vi "NanotecSMCPDDriver.set standby current.vi"(0 "VISA resource name":refnum<visa-resource-name>, 1 "contollerID":i32=-1, 3 "standbyCurrent [A]":dbl, 5 "error in (no error)":errorcluster) -> (14 "VISA resource name out":refnum<visa-resource-name>, 15 "contollerID out":i32=-1, 19 "error out":errorcluster)   [LabVIEW 2014, in "NanotecSMCPDDriver.lvlib"]
doc: "Sets the phase current of the motor that will be used in stand-by mode. This current will be applied when the motor is not moving."
uses:
  NanotecSMCPDDriver.lvlib
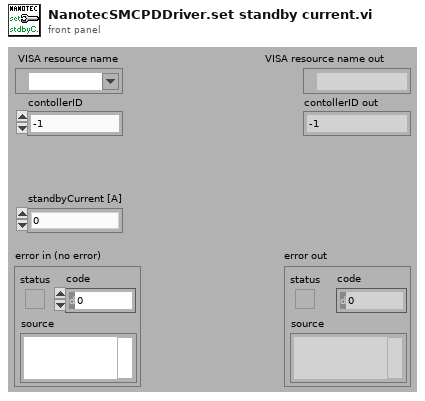
[diagram p1: front panel]
types:
  T1 = typedef "NanotecSMCPDDriver.lvlib/NanotecSMCPDDriver.hardware types.ctl" = enum16{"unknown", "PD4", "PD4Ic", "PD2Ic", "SMCI32", "SMCI47"}
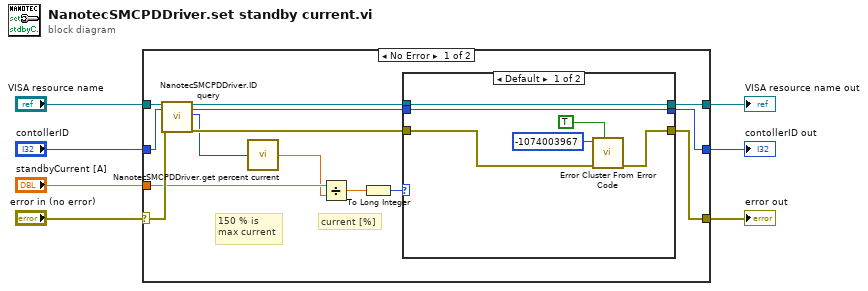
[diagram p0: block diagram]
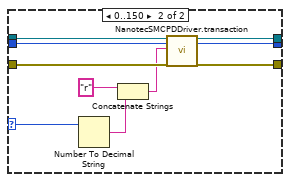
[diagram p2: hidden frame]
diagram:
  n1 = case shown="No Error" "error in (no error)" {
    selector: "error in (no error)" -> [w14 w38]
    tunnel: [w20 w40] -> w7
    tunnel: [w19 w38] -> w6
    tunnel: "VISA resource name" -> [w18 w40]
    tunnel: "contollerID" -> [w17 w39]
    tunnel: [w21 w39] -> w3
    tunnel: "standbyCurrent [A]" -> [w11 _]
    frame No Error {
      # "current [%]"
      # "150 % is\nmax current"
      n2 = call "NanotecSMCPDDriver.ID query.vi"("VISA resource name"=w18, "contollerID"=w17, "error in (no error)"=w14) -> ("VISA resource name out"=w15:refnum<visa-resource-name>, "contollerID out"=w16:i32, "hardwareType"=w12:T1, "error out"=w13:errorcluster)  [unwired: 12 in, 1 out]
      n3 = call "NanotecSMCPDDriver.get percent current.vi"("hardwareType"=w12) -> ("percentCurrent [A/%]"=w10:dbl)
      n4 = Divide(x=w11, y=w10) -> (x/y=w9:dbl)
      n5 = To Long Integer(number=w9) -> (32bit integer=w8:i32)
      n6 = case shown="Default" w8 {
        selector: w8 -> [_ w28]
        tunnel: w15 -> [w27 w37]
        tunnel: w16 -> [w22 w36]
        tunnel: [w22 w35] -> w21
        tunnel: [w27 w34] -> w20
        tunnel: [w26 w33] -> w19
        tunnel: w13 -> [w25 w32]
        frame Default {
          n7 = call <vilib>:"Error Cluster From Error Code.vi"("show call chain? (False)"=TRUE, "error in (no error)"=w25, "error code (0)"=-1074003967) -> ("error out"=w26:errorcluster)  [unwired: 6 in]
        }
        frame 0..150 {
          n8 = Number To Decimal String(number=w28) -> (decimal integer string=w31:string)  [unwired: 1 in]
          n9 = Concatenate Strings("r" ("commandString"), w31) -> (w29:string)
          n10 = call "NanotecSMCPDDriver.transaction.vi"("VISAresource"=w37, "contollerID"=w36, "commandString"=w29, "error in (no error)"=w32) -> ("VISAresource out"=w34:refnum<visa-resource-name>, "contollerID out"=w35:i32, "error out"=w33:errorcluster)  [unwired: 10 in, 3 out]
        }
      }
    }
    frame Error {
    }
  }
  "VISA resource name out" <- w7
  "error out" <- w6
  "contollerID out" <- w3
